vi "PiezoSignal.v2.vi"(4 "Microscope Settings in":T1={"Mode"=enum."X", "Slit"={"Scanning Mode"=0.0, "Slit Width /%"=0.0}, "Colour"=[], "Exposure/ms"=0.0, "Piezo Position /um"=0.0, "ROI"={"X"={"Start /px"=0.0, "Step /px"=0.0, "Range /px"=0.0}, "Y"={"Start /px"=0.0, "Step /px"=0.0, "Range /px"=0.0}, "Z "={"Start /um"=0.0, "Step/um"=0.0, "Range /um"=0.0}, "T "={"Start /s"=0.0, "Step /s"=1.0, "Range /s"=100.0}}, "Samples per millisecond"=0.0, "Relax/ms"=0.0, "Readout Direction"=0.0, "Trigger Source"=0.0, "Camera Delay /ms"=0.0, "Under Scan /ms"=0.0, "Calibration Coordinates"={"Top Left"=[-4.418670520231216, -0.1592138728323702, 10.0], "Top Right"=[-9.501965317919073, -0.1592138728323702, 10.0], "Bottom Left"=[-4.4508670520231215, 0.0, 0.0], "Bottom Right"=[-9.53757225433526, 0.0, 0.0], "Waveforms"={"Analogue Out"=[], "Digital Out"=[]}}} {"Under Scan /ms" min=0.0 max=10.0 step=0.05; "ROI"."T"."Range /s" min=0.0 max=10.0 step=0.05; "ROI"."T"."Step /s" min=0.0 max=10.0 step=0.05; "ROI"."T"."Start /s" min=0.0 max=10.0 step=0.05; "ROI"."X"."Range /px" min=0.0 max=10.0 step=0.05; "ROI"."X"."Step /px" min=0.0 max=10.0 step=0.05; "ROI"."X"."Start /px" min=0.0 max=10.0 step=0.05; "ROI"."Y"."Range /px" min=0.0 max=10.0 step=0.05; "ROI"."Y"."Step /px" min=0.0 max=10.0 step=0.05; "ROI"."Y"."Start /px" min=0.0 max=10.0 step=0.05; "ROI"."Z"."Range /um" min=0.0 max=10.0 step=0.05; "ROI"."Z"."Step/um" min=0.0 max=10.0 step=0.05; "ROI"."Z"."Start /um" min=0.0 max=10.0 step=0.05; "Colour"."Filter" items=["Empty"=1, ""=2, ""=3, "561"=4, ""=5, "488"=6]; "Camera Delay /ms" min=0.0 max=10.0 step=0.05; "Trigger Source" items=["Internal"=1.0, "External"=2.0]; "Readout Direction" items=["Forward"=1.0, "Backward"=2.0]; "Slit"."Scanning Mode" items=["Full Frame"=1.0, "Slit Scanning"=12.0]; "Piezo Position /um" min=0.0 max=10.0 step=0.05}) -> (1 "Piezo Signal":dbl[](graph))   [LabVIEW 2016]
uses:
  controls/Microscope Settings.ctl
  <vilib>/Analysis/NI_AALBase.lvlib
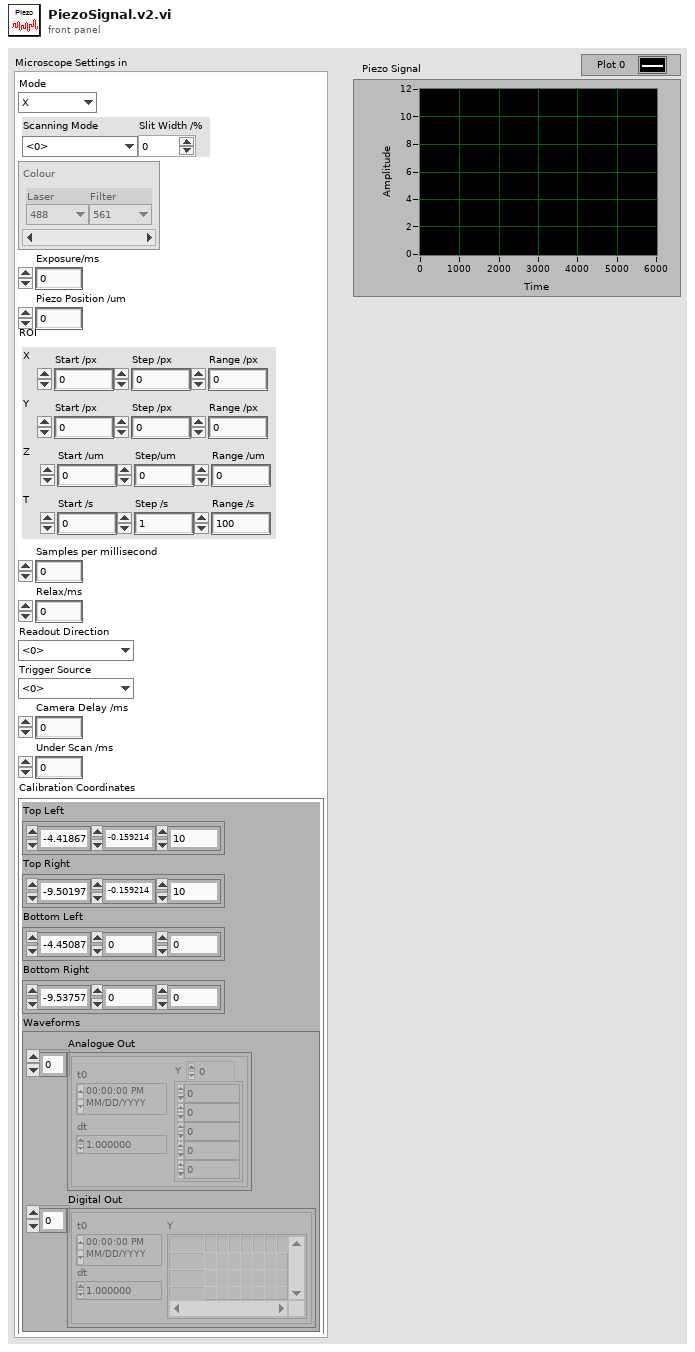
[diagram p1: front panel]
types:
  T1 = typedef "Microscope Settings.ctl" = cluster{"Mode":enum16{"Brightfield", "X", "XY", "XYZ", "XYZT", "XYZC", "Tweezers", "Virus"}, "Slit":cluster{"Scanning Mode":dbl, "Slit Width /%":dbl}, "Colour":cluster{"Laser":enum16{"Brightfield", "445", "488", "561", "647"}, "Filter":u16}[], "Exposure/ms":dbl, "Piezo Position /um":dbl, "ROI":cluster{"X":cluster{"Start /px":dbl, "Step /px":dbl, "Range /px":dbl}, "Y":cluster{"Start /px":dbl, "Step /px":dbl, "Range /px":dbl}, "Z ":cluster{"Start /um":dbl, "Step/um":dbl, "Range /um":dbl}, "T ":cluster{"Start /s":dbl, "Step /s":dbl, "Range /s":dbl}}, "Samples per millisecond":dbl, "Relax/ms":dbl, "Readout Direction":dbl, "Trigger Source":dbl, "Camera Delay /ms":dbl, "Under Scan /ms":dbl, "Calibration Coordinates":cluster{"Top Left":dbl[], "Top Right":dbl[], "Bottom Left":dbl[], "Bottom Right":dbl[], "Waveforms":cluster{"Analogue Out":waveform(dbl)[], "Digital Out":digitalwaveform[]}}}
  T2 = enum16{"Brightfield", "X", "XY", "XYZ", "XYZT", "XYZC", "Tweezers", "Virus"}
  T3 = cluster{"Start /um":dbl, "Step/um":dbl, "Range /um":dbl}
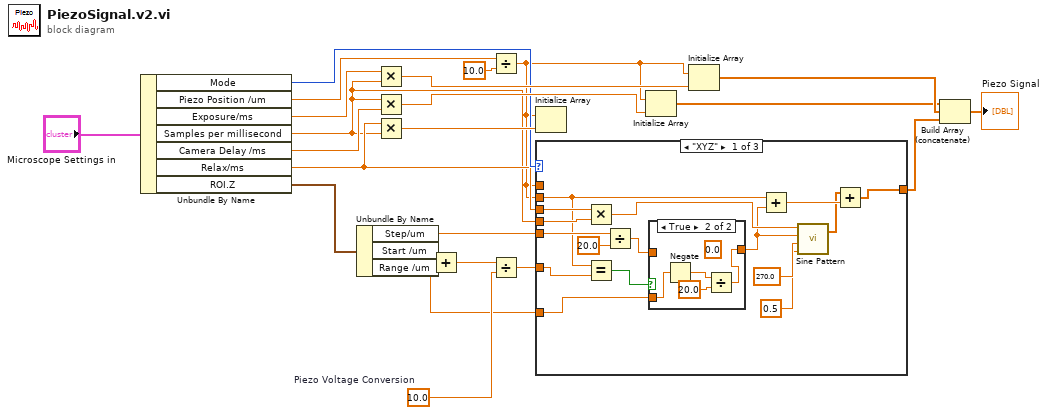
[diagram p0: block diagram]
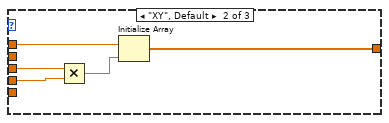
[diagram p3: hidden frame]
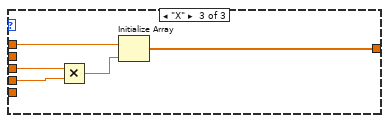
[diagram p4: hidden frame]
diagram:
  w3 = 10.0  # Piezo Voltage Conversion
  n1 = Unbundle By Name("Microscope Settings in") -> ("Mode"=w11:T2, "Piezo Position /um"=w12:dbl, "Exposure/ms"=w16:dbl, "Samples per millisecond"=w9:dbl, "Camera Delay /ms"=w15:dbl, "Relax/ms"=w10:dbl, "ROI.Z"=w14:T3)
  n2 = Unbundle By Name(w14) -> ("Step/um"=w8:dbl, "Start /um"=w5:dbl, "Range /um"=w1:dbl)
  n3 = Multiply(x=w16, y=w9) -> (x*y=w22:dbl)
  n4 = Multiply(x=w9, y=w15) -> (x*y=w18:dbl)
  n5 = Multiply(x=w10, y=w9) -> (x*y=w13:dbl)
  n6 = Add(x=w5, y=w1) -> (x+y=w4:dbl)
  n7 = Divide(x=w12, y=10.0) -> (x/y=w7:dbl)
  n8 = Divide(x=w4, y=w3) -> (x/y=w2:dbl)
  n9 = Initialize Array(w7, w13) -> ()  [unwired: 1 out]
  n10 = case shown="\"XYZ\"" w11 {
    tunnel: w7 -> [_ w48 w53]
    tunnel: w10 -> [w34 w47 w52]
    tunnel: w9 -> [w35 w46 w51]
    tunnel: [w31 w45 w50] -> w6
    tunnel: w8 -> [w36 _ _]
    tunnel: w7 -> [w28 _ _]
    tunnel: w2 -> [w27 _ _]
    tunnel: w1 -> [w24 _ _]
    frame "XYZ" {
      n11 = Multiply(x=w34, y=w35) -> (x*y=w33:dbl)
      n12 = Equal?(x=w28, y=w27) -> (x = y?=w29:bool)
      n13 = Divide(x=w36, y=20.0 ("phase(degrees)")) -> (x/y=w26:dbl)
      n14 = case shown="True" w29 {
        tunnel: w26 -> [w40 _]
        tunnel: [w40 w41] -> w25
        tunnel: w24 -> [_ w44]
        frame False {
        }
        frame True {
          (unwired) 0.0 ("phase(degrees)")
          n15 = Negate(x=w44) -> (-x=w42:dbl)
          n16 = Divide(x=w42, y=20.0) -> (x/y=w41:dbl)
        }
      }
      n17 = Add(x=w28, y=w25) -> (x+y=w37:dbl)
      n18 = call <vilib>:"Sine Pattern.vi"("cycles"=0.5, "phase(degrees)"=270.0, "amplitude"=w25, "samples"=w33) -> ("Sinusoidal Pattern"=w32:dbl[])  [unwired: 1 out]
      n19 = Add(x=w32, y=w37) -> (x+y=w31:dbl[])
    }
    frame "XY", Default {
      n20 = Multiply(x=w47, y=w46) -> (x*y=w49:dbl)
      n21 = Initialize Array(w48, w49) -> (w45:dbl[])
    }
    frame "X" {
      n22 = Multiply(x=w52, y=w51) -> (x*y=w54:dbl)
      n23 = Initialize Array(w53, w54) -> (w50:dbl[])
    }
  }
  n24 = Initialize Array(w7, w18) -> (w19:dbl[])
  n25 = Initialize Array(w7, w22) -> (w21:dbl[])
  n26 = Build Array (concatenate)(w19, w21, w6) -> (→"Piezo Signal":dbl[])
